vi "getNewValueFromXml.vi"(8 "error in (no error)":errorcluster, 10 "Xml":refnum<class "xmlNode.lvclass">, 11 "SingleToneRamp in":refnum<class "SingleToneRamp.lvclass">) -> (0 "error out":errorcluster, 2 "Xml out":refnum<class "xmlNode.lvclass">, 3 "SingleToneRamp out":refnum<class "SingleToneRamp.lvclass">)   [LabVIEW 2009, in "Tools.lvlib" / "Scripting.lvlib" / "SingleToneRamp.lvclass"]
uses:
  SingleToneRamp.lvclass
  xmlNode/xmlNode.lvclass
  ScriptEvent.lvclass
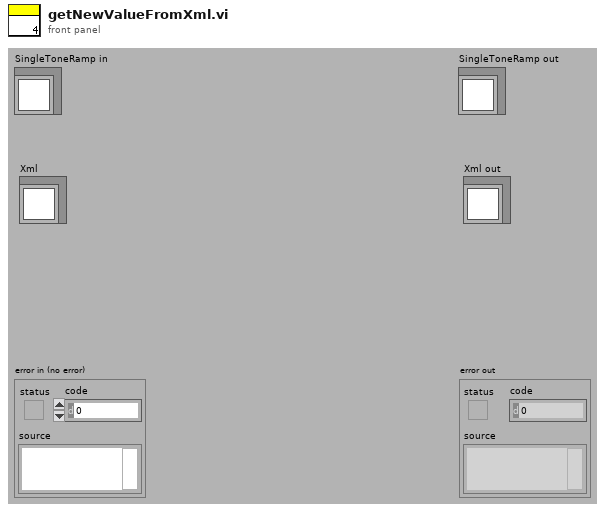
[diagram p1: front panel]
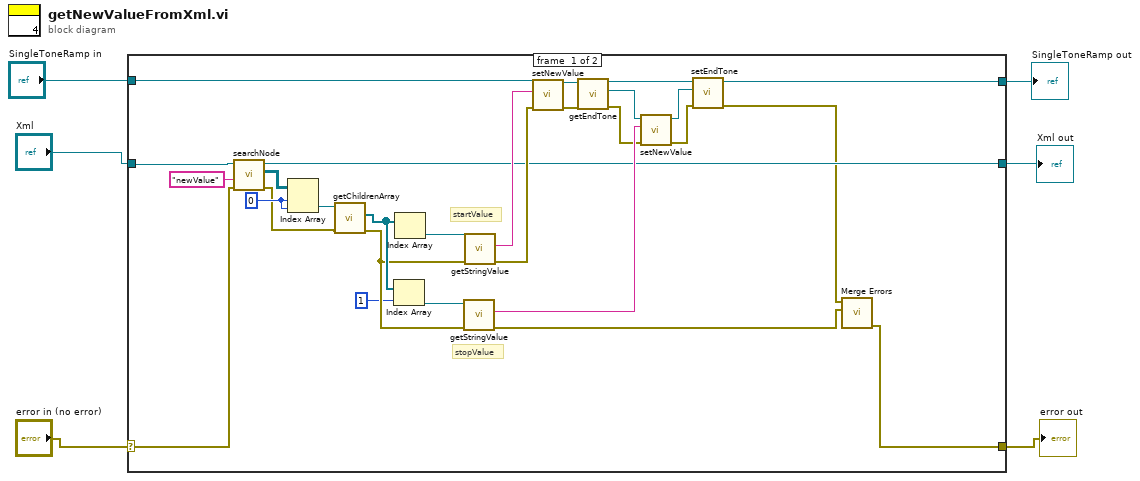
[diagram p0: block diagram]
diagram:
  n1 = case shown="No Error" "error in (no error)" {
    selector: "error in (no error)" -> [w19 w35]
    tunnel: "SingleToneRamp in" -> [w24 w36]
    tunnel: [w8 w36] -> w5
    tunnel: "Xml" -> [w31 w37]
    tunnel: [w18 w35] -> w2
    tunnel: [w17 w37] -> w1
    frame #0 {
      w32 = 0
      # "stopValue"
      # "startValue"
      n2 = call-dynamic "searchNode.vi"("error in (no error)"=w19, "searchElementName"="newValue", "xmlNode in"=w31) -> ("error out"=w29:errorcluster, "arrayXmlNodes"=w33:refnum<class "xmlNode.lvclass">[][], "xmlNode out"=w17:refnum<class "xmlNode.lvclass">)  [unwired: 6 in]
      n3 = Index Array(array=w33, index (row)=w32, index (col)=w32) -> (element=w30:refnum<class "xmlNode.lvclass">)
      n4 = call-dynamic "getChildrenArray.vi"("error in (no error)"=w29, "xmlNode.lvclass in"=w30) -> ("error out"=w25:errorcluster, "Children"=w28:refnum<class "xmlNode.lvclass">[])  [unwired: 7 in, 1 out]
      n5 = Index Array(array=w28, index=1) -> (element=w26:refnum<class "xmlNode.lvclass">)
      n6 = Index Array(array=w28) -> (element=w27:refnum<class "xmlNode.lvclass">)  [unwired: 1 in]
      n7 = call-dynamic "getStringValue.vi"("error in (no error)"=w25, "xmlNode.lvclass in"=w26) -> ("error out"=w20:errorcluster, "stringValue"=w21:string)  [unwired: 7 in, 1 out]
      n8 = call-dynamic "getStringValue.vi"("error in (no error)"=w25, "xmlNode.lvclass in"=w27) -> ("error out"=w22:errorcluster, "stringValue"=w23:string)  [unwired: 7 in, 1 out]
      n9 = call "setNewValue.vi"("error in (no error)"=w22, "newValue"=w23, "ScriptEvent.lvclass in"=w24) -> ("error out"=w14:errorcluster, "ScriptEvent.lvclass out"=w15:refnum<class "SingleToneRamp.lvclass">)  [unwired: 7 in]
      n10 = call "getEndTone.vi"("error in (no error)"=w14, "SingleToneRamp.lvclass in"=w15) -> ("error out"=w13:errorcluster, "endTone"=w12:refnum<class "SingleTone.lvclass">, "SingleToneRamp.lvclass out"=w11:refnum<class "SingleToneRamp.lvclass">)  [unwired: 7 in]
      n11 = call "setNewValue.vi"("error in (no error)"=w13, "newValue"=w21, "ScriptEvent.lvclass in"=w12) -> ("error out"=w9:errorcluster, "ScriptEvent.lvclass out"=w10:refnum<class "SingleTone.lvclass">)  [unwired: 7 in]
      n12 = call "setEndTone.vi"("error in (no error)"=w9, "EndTone"=w10, "SingleToneRamp.lvclass in"=w11) -> ("error out"=w7:errorcluster, "SingleToneRamp.lvclass out"=w8:refnum<class "SingleToneRamp.lvclass">)  [unwired: 7 in]
      n13 = call <vilib>:"Merge Errors.vi"("error in 2 (no error)"=w20, "error in 1 (no error)"=w7) -> ("error out"=w18:errorcluster)  [unwired: 5 in]
    }
    frame #1 {
    }
  }
  "error out" <- w2
  "SingleToneRamp out" <- w5
  "Xml out" <- w1
